vi "NI 5772 (AC) - TIS Mode Enabled (Host)_Copy.vi"() -> ()   [LabVIEW 2020]
doc: "Example Description:\nThis example demonstrates how to enable Time Interleaved Sampling with the NI 5772 adapter module to achieve a sampling rate of 1.6GS/s. This example continuously acquires records of analog input data from the NI 5772 adapter module. It allows you to select an AI channel, trigger type, and record size. This VI must be compiled before it is run. \n\nVI Configuration:\nThis example uses the NI PXI-7952R as the FPGA target by default. If you are using another FPGA target, complete the following steps to configure the host VI to use a VI configured for your FPGA target:\n1. On the block diagram, right-click the Open FPGA VI Reference (NI PXI-7952R) function and select Configure Open FPGA VI Reference.\n2. Browse for a new target by clicking the Browse Project button in the Open VI section.\n3. Select the VI under the target that matches your device. Click OK to select this VI.\n4. Click OK to exit the dialog box and to apply the new selection to the FPGA VI.\n5. Save the VI.\n\nRunning the VI:\n1. Select a RIO Resource that corresponds to the FPGA device configured above.\n2. Clock Configuration: Select the desired clock source for the adapter module.\nAnalog Input: Configure the AI Channel, Record Size, and Trigger Type controls. If you are using the analog trigger type, configure the Trigger Level (V) control.\n3. Click the run arrow to run the VI.\n4. If the Trigger Type is set to Software, click the Software Trigger button to acquire a single record of data. If the Trigger Type is set to Data Edge, a record of data is acquired each time the input signal rises above the trigger level.\n\nThe Record Size, Trigger Type, and Trigger Level (V) controls can all be configured while the VI is running. \n\nNote: The AI Channel control must be configured before the VI is run.\n\nExecution Steps:s\n1. Open a session to the FPGA VI and run the VI.\n2. Wait for the adapter module to load its default configuration.\n3. Configure the NI 5772 for Time Interleaved Sampling (TIS)\n4. The Trigger type and record size for a single record acquisition are configured.\n5. Based on the trigger type, either wait for the software trigger Boolean to assert or configure the desired trigger level and arm the trigger.\n6. After the trigger is armed, a single record of data is acquired and read.\n7. Stop the VI when the stop button is pressed or when an error has occurred. \n8. Close the FPGA VI reference and display any errors."
uses:
  <vilib>/rvi/interface/nirviReadWriteControl/nirviReadWriteControl.xnode
  <vilib>/rvi/interface/nirviMethod/nirviMethod.xnode
  <vilib>/rvi/interface/nirviCloseFPGA/nirviCloseFPGA.xnode
  <vilib>/rvi/interface/nirviOpenFPGA/nirviOpenFPGA.xnode
  <vilib>/rvi/errors/niLvFpgaAdjustHostInterfaceError.vi
  NiFpgaLv.dll
  <vilib>/Utility/error.llb/Error Cluster From Error Code.vi
  <vilib>/rvi/interface/Simulation/niFpgaSimulationCallBeginRW.vi
  <vilib>/FPGAPlugInAG/Dynamic/niLvFpga_ReadFifo_Dynamic.vi
  <vilib>/rvi/errors/niLvFpgaMergeErrorWithErrorCode.vi
  FPGA Bitfiles/acoustoxv3_FPGATarget_OriginalDigitize_EOlkFE5eWpM.lvbitx
  Digi/OriginalDigitizerLive.vi
  <vilib>/FPGAPlugInAG/PXIe-7962R/niLvFpga_Open_PXIe-7962R.vi
  <vilib>/rvi/interface/common/dynamic/niFpgaDynamicAddResources.vi
  <vilib>/FPGAPlugInAG/Dynamic/niLvFpga_Close_Dynamic.vi
  <vilib>/userdefined/High Color/nirio_resource_hc.ctl
  Digi/Controls/TIS Mode.ctl
panel:
  in  "DS":u8
  out "Elements Remaining":u32
  out "Requested":u16
  in  "TIS Mode":T1=1 items=["TIS Mode (CH0 Only)"=1, "TIS Mode (CH1 Only)"=2, "Dual TIS Mode (CH0 and CH1)"=3]
  out "TIS Configured?":bool
  out "Analog Input":cluster{"Start Time":dbl, dbl, ext[]}(graph) caption="Acquired Waveform"
  out "error out":errorcluster
  in  "stop":bool
  in  "Trigger Level (V)":dbl
  in  "Software Trigger":bool
  in  "Record Size":u16=1024
  in  "Trigger Type":enum8{"Software", "Data Edge"}(ring)
  in  "RIO Resource":T2="RIO0"
  out "Configured?":bool
  # "Resource Configuration"
  # "AI Configuration"
  # "For instructions, select Help>>Show Context Help and move the cursor over the VI icon to display help for this VI."
  # "Interleaved Configuration"
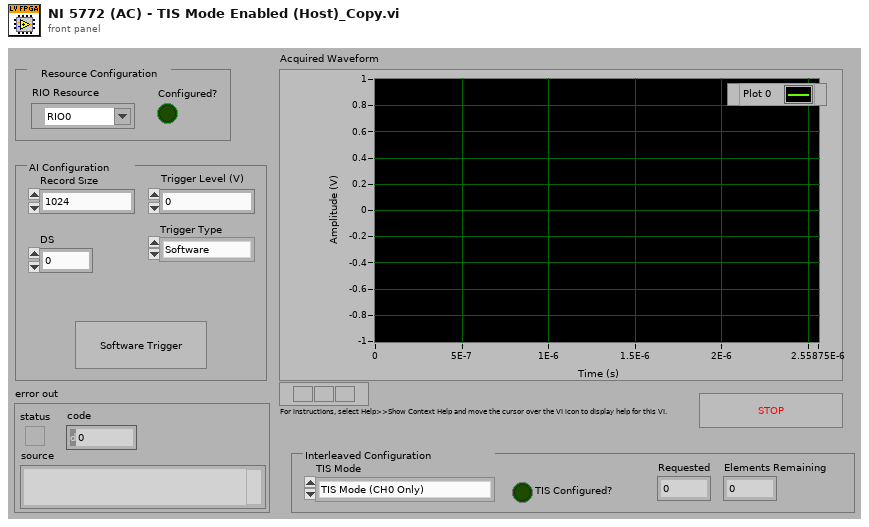
[diagram p1: front panel]
types:
  T1 = typedef "TIS Mode.ctl" = u16
  T2 = typedef "nirio_resource_hc.ctl" = tag
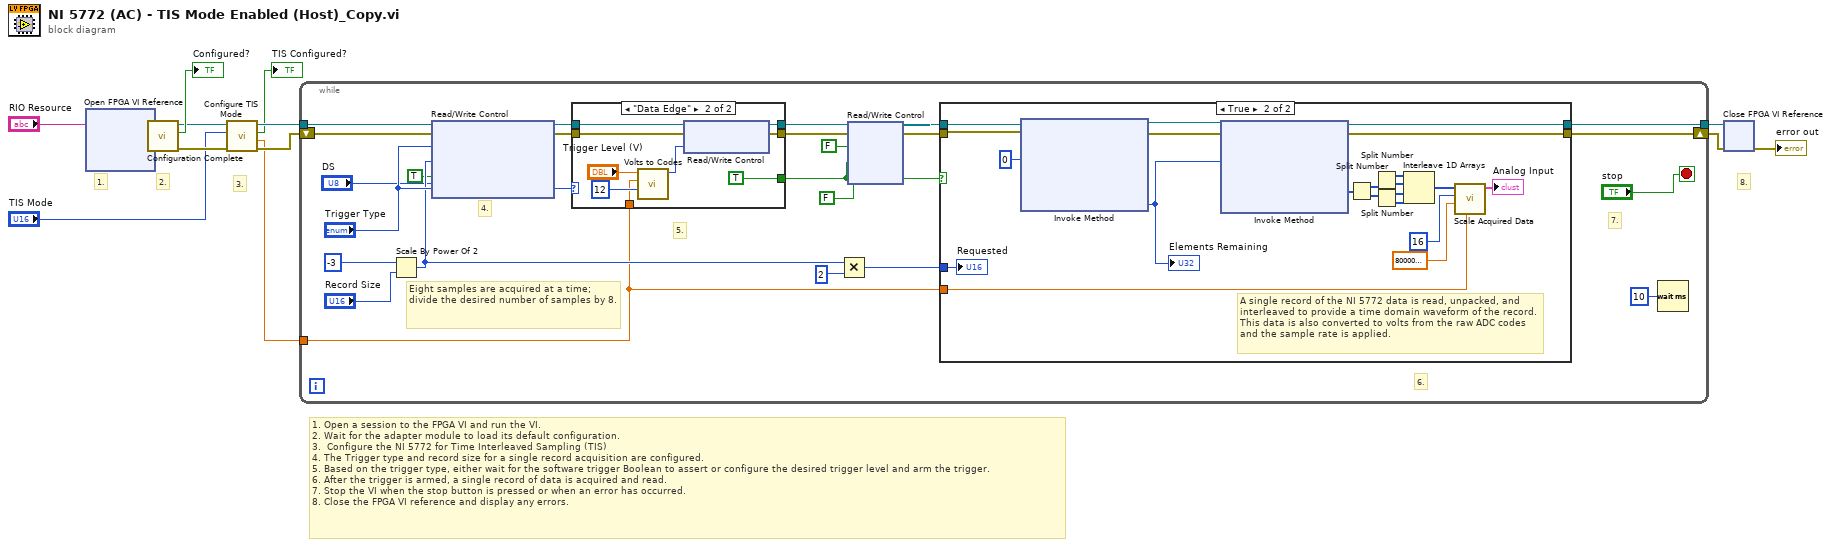
[diagram p0: block diagram]
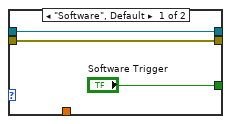
[diagram p3: hidden frame]
diagram:
  # "8."
  # "3."
  # "2."
  # "1."
  # "1. Open a session to the FPGA VI and run the VI.\n2. Wait for the adapter module to load its default configuration.\n3.  Configure the NI 5772 for Time Interleaved Sampling (TIS)\n4. The Trigger type and record size for a single record acquisition are configured.\n5. Based on the trigger type, either wait for the software trigger Boolean to assert or configure the desired trigger level and arm the trigger.\n6. After the trigger is armed, a single record of data is acquired and read.\n7. Stop the VI when the stop button is pressed or when an error has occurred.  \n8. Close the FPGA VI reference and display any errors."
  n1 = xnode "Open FPGA VI Reference"("resource name"="RIO Resource") -> ("FPGA VI Reference Out"=w1:refnum<k20>, "error out"=w10:errorcluster)  [unwired: 1 in]
  n2 = call "Configuration Complete.vi"("error in"=w10, "FPGA VI Reference In"=w1) -> ("error out"=w9:errorcluster, "Configured?"=→"Configured?":bool, "FPGA VI Reference Out"=w7:refnum<k20>)  [unwired: 7 out]
  n3 = call "Configure TIS Mode.vi"("error in"=w9, "TIS Mode"="TIS Mode", "FPGA VI Reference In"=w7) -> ("error out"=w8:errorcluster, "range (Vpp)"=w2:dbl, "TIS Configured?"=→"TIS Configured?":bool, "FPGA VI Reference Out"=w6:refnum<k20>)  [unwired: 5 in]
  n4 = while {
    tunnel: [w37] -> w13
    tunnel: w6 -> [w29]
    shift-right: [w32] -> w11
    shift-left: w8 -> [w28]
    tunnel: w2 -> [w23]
    stop <- "stop" stop-if-true
    # "7."
    # "Eight samples are acquired at a time; divide the desired number of samples by 8."
    # "6."
    # "5."
    # "4."
    n5 = Scale By Power Of 2(n=-3, x="Record Size") -> (x*2^n=w24:u16)
    n6 = xnode "Read/Write Control"("FPGA VI Reference In"=w29, "error in"=w28, "Trigger Type"="Trigger Type", "Samples Per Trigger"=w24, "Arm Trigger"=TRUE, "DS"="DS") -> ("FPGA VI Reference Out"=w31:refnum<k20>, "error out"=w30:errorcluster)
    n7 = case shown="\"Data Edge\"" "Trigger Type" {
      tunnel: w31 -> [w64 w73]
      tunnel: w30 -> [w63 w72]
      tunnel: [w64 w71] -> w36
      tunnel: [w63 w70] -> w35
      tunnel: ["Software Trigger" TRUE ("Acquire")] -> w19
      tunnel: w23 -> [_ w65]
      frame "Software", Default {
      }
      frame "Data Edge" {
        n8 = call "Volts to Codes.vi"("Number of Bits"=i16 12, "range (Vpp)"=w65, "Data In"="Trigger Level (V)") -> ("Data Out"=w66:i16)  [unwired: 8 out]
        n9 = xnode "Read/Write Control"("FPGA VI Reference In"=w73, "error in"=w72, "Trigger Level"=w66) -> ("FPGA VI Reference Out"=w71:refnum<k20>, "error out"=w70:errorcluster)
      }
    }
    n10 = Multiply(x=w24, y=u16 2) -> (x*y=w22:u16)
    n11 = xnode "Read/Write Control"("FPGA VI Reference In"=w36, "error in"=w35, "Trigger"=FALSE, "Trigger"=w19, "Trigger"=FALSE) -> ("FPGA VI Reference Out"=w34:refnum<k20>, "error out"=w33:errorcluster)
    n12 = case shown="True" w19 {
      tunnel: w34 -> [w39 w43]
      tunnel: w33 -> [w40 w44]
      tunnel: [w40 w61] -> w32
      tunnel: [w39 w60] -> w37
      tunnel: w22 -> [_ w47]
      tunnel: w23 -> [_ w56]
      frame False {
      }
      frame True {
        # "A single record of the NI 5772 data is read, unpacked, and interleaved to provide a time domain waveform of the record. This data is also converted to volts from the raw ADC codes and the sample rate is applied."
        n13 = xnode "Invoke Method"("FPGA VI Reference In"=w43, "error in"=w44, "Number of Elements"=u32 0) -> ("FPGA VI Reference Out"=w46:refnum<k20>, "error out"=w45:errorcluster, "Elements Remaining"=w42:u32)  [unwired: 1 in, 1 out]
        "Elements Remaining" <- w42
        n14 = xnode "Invoke Method"("FPGA VI Reference In"=w46, "error in"=w45, "Number of Elements"=w42) -> ("FPGA VI Reference Out"=w60:refnum<k20>, "error out"=w61:errorcluster, "Data"=w55:u64[])  [unwired: 1 in, 1 out]
        n15 = Split Number(x=w55) -> (hi(x)=w54:u32[], lo(x)=w53:u32[])
        n16 = Split Number(x=w54) -> (hi(x)=w51:u16[], lo(x)=w48:u16[])
        n17 = Split Number(x=w53) -> (hi(x)=w49:u16[], lo(x)=w50:u16[])
        n18 = Interleave 1D Arrays(w51, w48, w49, w50) -> (w52:u16[])
        n19 = call "Scale Acquired Data.vi"("range (V)"=w56, "Sample Rate"=800000000.0, "Number of Bits"=i16 16, "Data In"=w52) -> ("output waveform"=→"Analog Input":cluster{"Start Time":dbl, dbl, ext[]})  [unwired: 1 in, 6 out]
        "Requested" <- w47
      }
    }
    n20 = Wait (ms)(milliseconds to wait=u32 10) -> ()  [unwired: 1 out]
  }
  n21 = xnode "Close FPGA VI Reference"("FPGA VI Reference In"=w13, "error in"=w11) -> ("error out"=→"error out":errorcluster)
